vi "git_commit-m.vi"(8 "Error In":errorcluster, 9 "commit message":string, 10 "Working Directory In":path=path "", 11 "commit_button":bool) -> (0 "Error Out":errorcluster, 1 "git commit output":string, 2 "Working Directory Out":path, 3 "commit_indicator":bool)   [LabVIEW 2026]
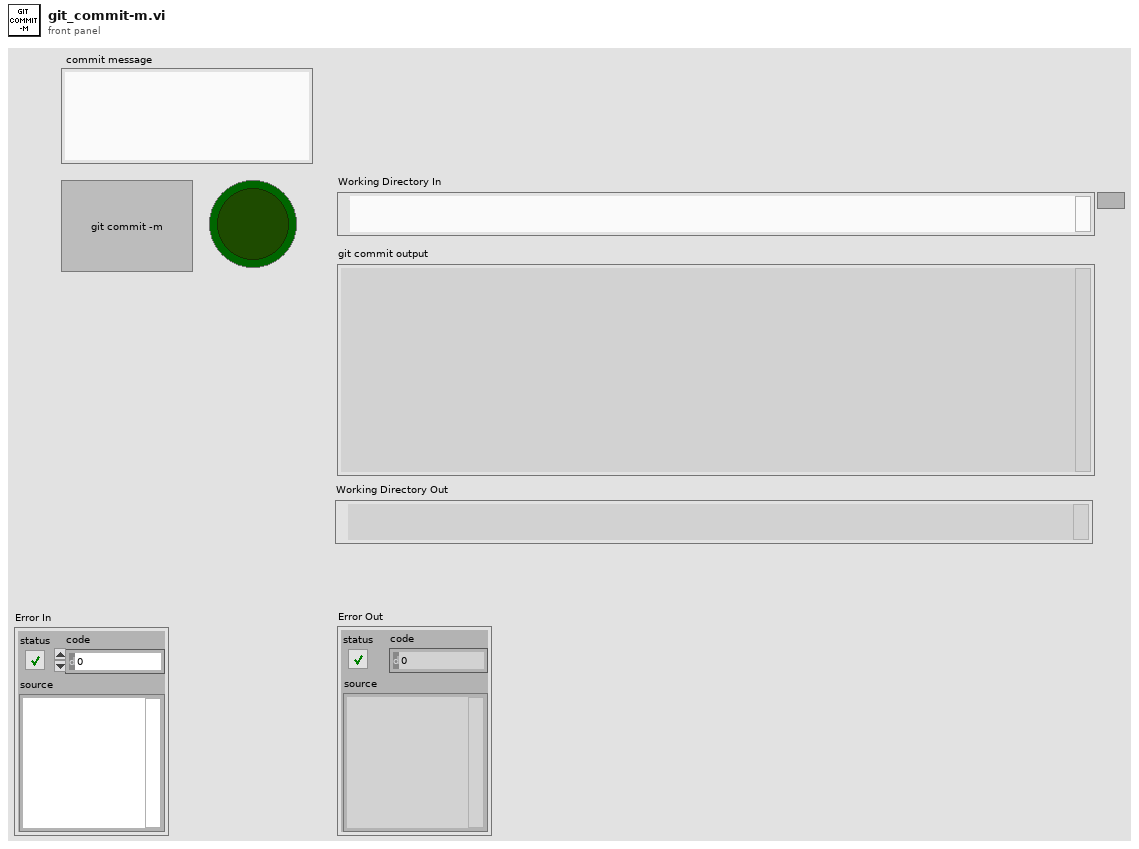
[diagram p1: front panel]
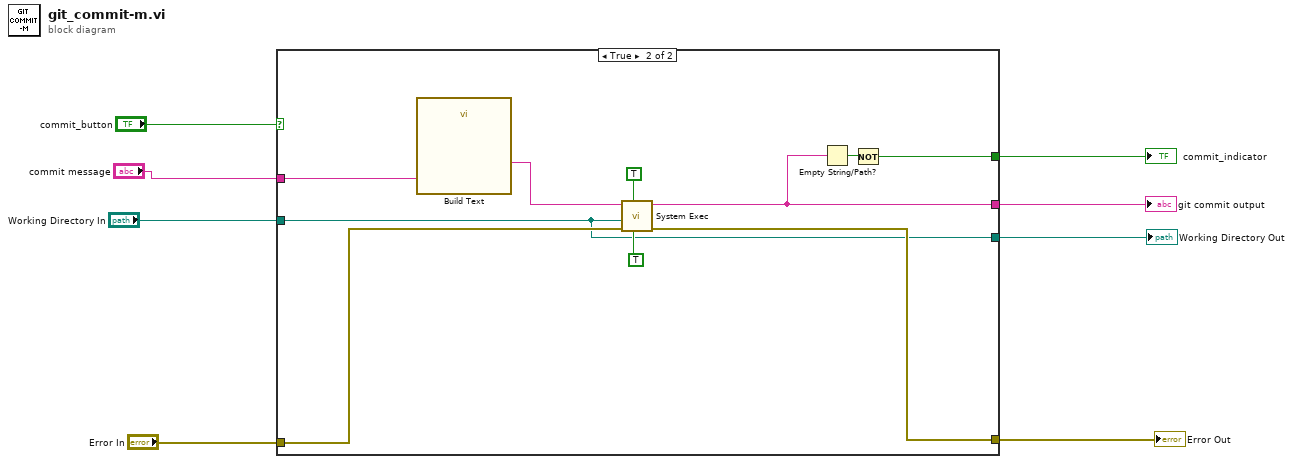
[diagram p0: block diagram]
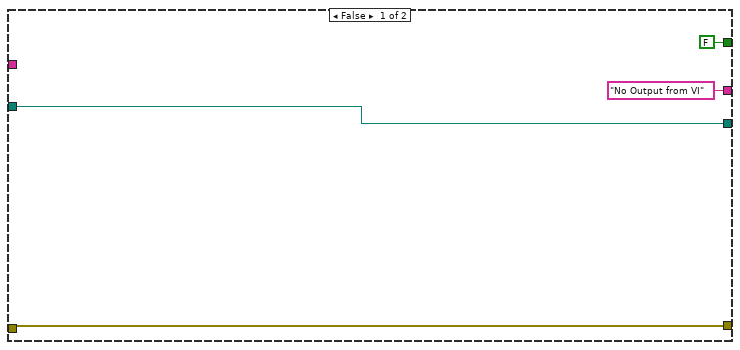
[diagram p2: hidden frame]
diagram:
  n1 = case shown="True" "commit_button" {
    tunnel: "Working Directory In" -> [w9 w13]
    tunnel: "Error In" -> [w10 w22]
    tunnel: [w10 w21] -> w6
    tunnel: ["No Output from VI" ("standard output") w19] -> w5
    tunnel: [FALSE w17] -> w4
    tunnel: "commit message" -> [_ w14]
    tunnel: [w9 w13] -> w1
    frame False {
    }
    frame True {
      n2 = call "Build Text"("commit message"=w14) -> ("Result"=w15:string)  [unwired: 13 in, 1 out]
      n3 = call <vilib>:"System Exec.vi"("run minimized? (F)"=TRUE, "wait until completion? (T)"=TRUE, "error in (no error)"=w22, "working directory"=w13, "command line"=w15) -> ("error out"=w21:errorcluster, "standard output"=w19:string)  [unwired: 3 in, 2 out]
      n4 = Empty String/Path?(string/path=w19) -> (empty?=w18:bool)
      n5 = Not(x=w18) -> (.not. x?=w17:bool)
    }
  }
  "Error Out" <- w6
  "git commit output" <- w5
  "commit_indicator" <- w4
  "Working Directory Out" <- w1
